vi "Ritter Dry Meter Calculations.vi"(0 "Heise Barometric Pressure (inHG)":dbl, 1 "Gas Temperature (F)":dbl, 2 "standardPressure (in HG)":dbl=30.0, 5 "Gas Pressure (in WC)":dbl, 7 "Gas Flow Rate (cuft/hr)-Uncorrected":dbl, 9 "Totalized Flow (cuft)-Uncorrected":dbl, 11 "error in (no error)":errorcluster, 12 "Gross Heating Value, Vol (Real, Dry)":dbl) -> (3 "CFdry":dbl, 4 "tempCorrectionFactor":dbl, 6 "pressureCorrectionFactor":dbl, 8 "gasFlowRate":dbl, 10 "gasVolume":dbl, 13 "btuEnergy":dbl, 14 "btuRate":dbl, 15 "error out":errorcluster)   [LabVIEW 2023]
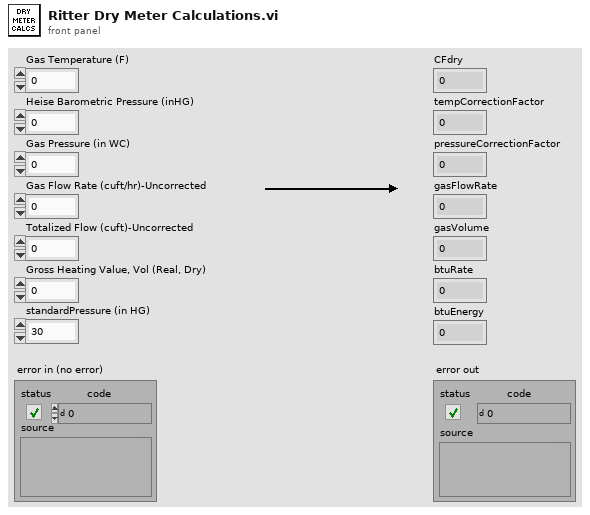
[diagram p1: front panel]
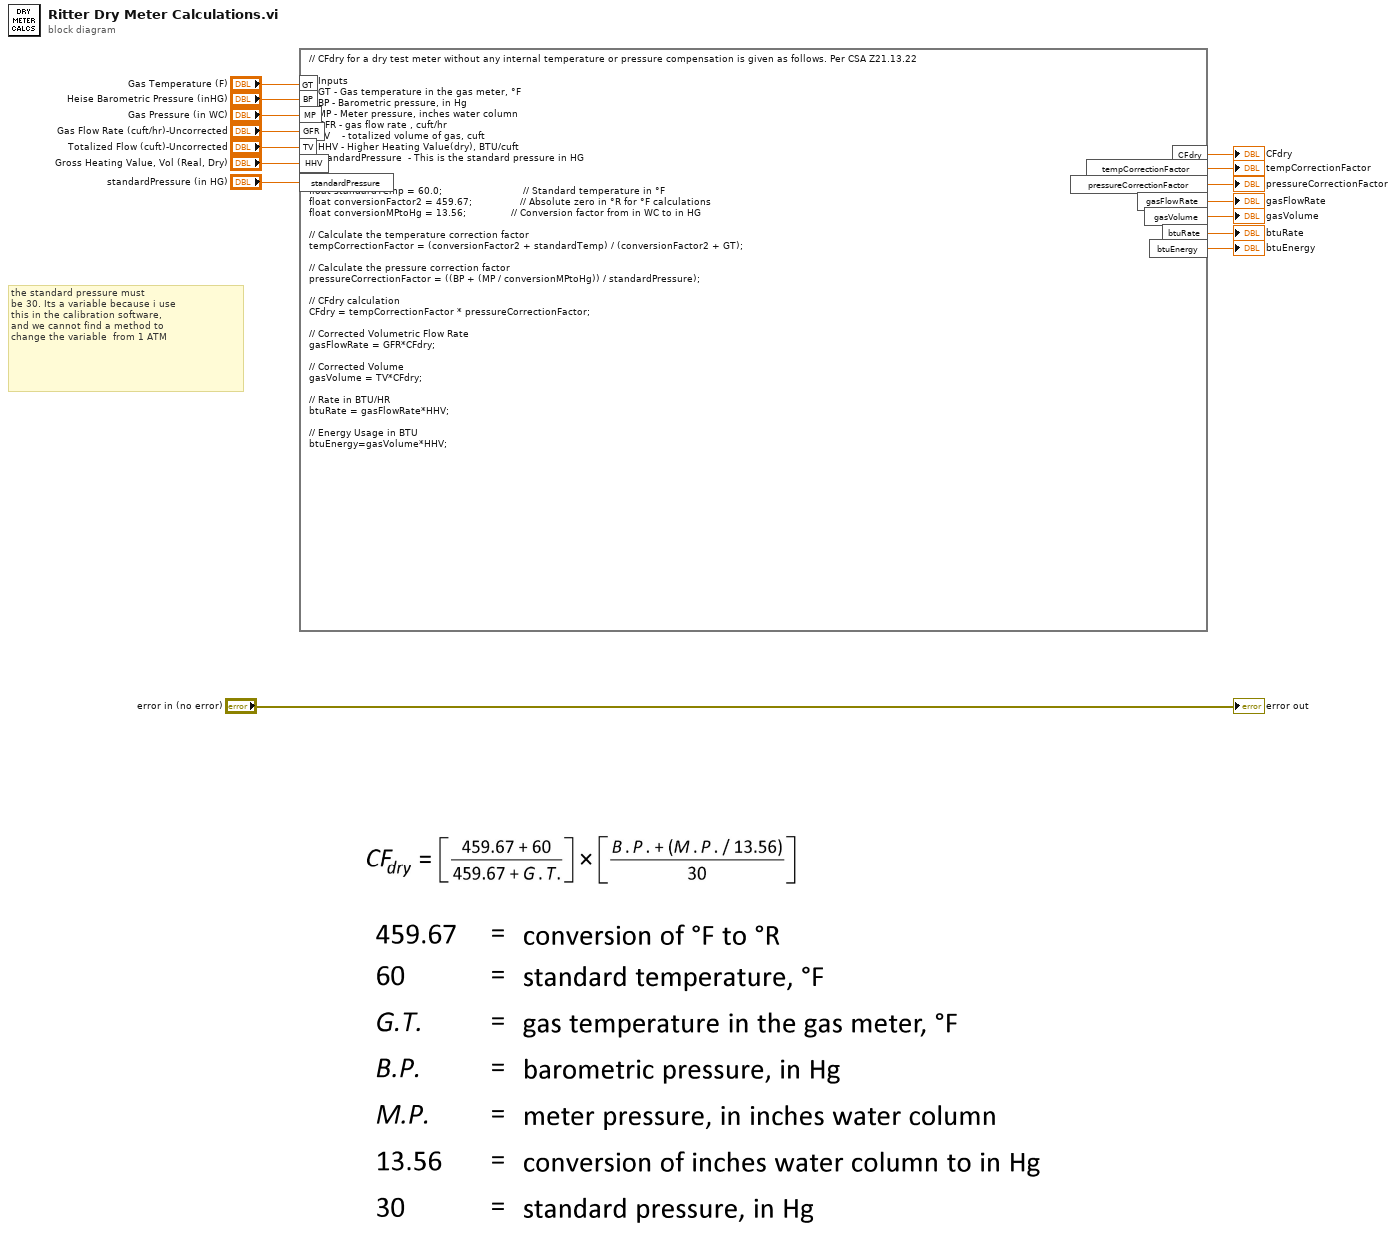
[diagram p0: block diagram]
diagram:
  # "the standard pressure must\nbe 30. Its a variable because i use\nthis in the calibration software, \nand we cannot find a method to\nchange the variable  from 1 ATM"
  n1 = formula code="// CFdry for a dry test meter without any internal temperature or pressure compensation is given as follows. Per CSA Z21.13.22   \n\n// Inputs\n// GT - Gas temperature in the gas meter, °F\n// BP - Barometric pressure, in Hg\n// MP - Meter pressure, inches water column\n// GFR - gas flow rate , cuft/hr\n// TV    - totalized volume of gas, cuft\n// HHV - Higher Heating Value(dry), BTU/cuft\n// standardPressure  - This is the standard pressure in HG\n\n// Constants\nfloat standardTemp = 60.0;                           // Standard temperature in °F\nfloat conversionFactor2 = 459.67;                // Absolute zero in °R for °F calculations\nfloat conversionMPtoHg = 13.56;               // Conversion factor from in WC to in HG\n\n// Calculate the temperature correction factor\ntempCorrectionFactor = (conversionFactor2 + standardTemp) / (conversionFactor2 + GT);\n\n// Calculate the pressure correction factor\npressureCorrectionFactor = ((BP + (MP / conversionMPtoHg)) / standardPressure);\n\n// CFdry calculation\nCFdry = tempCorrectionFactor * pressureCorrectionFactor;\n\n// Corrected Volumetric Flow Rate\ngasFlowRate = GFR*CFdry;\n\n// Corrected Volume\ngasVolume = TV*CFdry;\n\n// Rate in BTU/HR\nbtuRate = gasFlowRate*HHV;\n\n// Energy Usage in BTU\nbtuEnergy=gasVolume*HHV;"("GT"="Gas Temperature (F)", "BP"="Heise Barometric Pressure (inHG)", "MP"="Gas Pressure (in WC)", "GFR"="Gas Flow Rate (cuft/hr)-Uncorrected", "TV"="Totalized Flow (cuft)-Uncorrected", "HHV"="Gross Heating Value, Vol (Real, Dry)", "standardPressure"="standardPressure (in HG)") -> ("CFdry"=→"CFdry":dbl, "tempCorrectionFactor"=→"tempCorrectionFactor":dbl, "pressureCorrectionFactor"=→"pressureCorrectionFactor":dbl, "gasFlowRate"=→"gasFlowRate":dbl, "gasVolume"=→"gasVolume":dbl, "btuRate"=→"btuRate":dbl, "btuEnergy"=→"btuEnergy":dbl)
  "error out" <- "error in (no error)"
